vi "COMI PG Change Freq.vi"(9 "freq":dbl, 10 "ch":i32, 11 "hDevice":u32) -> (2 "function return":dbl, 3 "hDevice out":u32)   [LabVIEW 2017, in "Comidll.lvlib"]
doc: "double (COMI_PG_ChangeFreq) (HANDLE hDevice, int ch, double freq);"
uses:
  <userlib>/Comidll/Comidll.lvlib
  <userlib>/Comidll/Comidll.dll
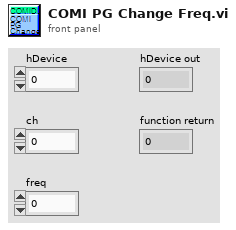
[diagram p1: front panel]
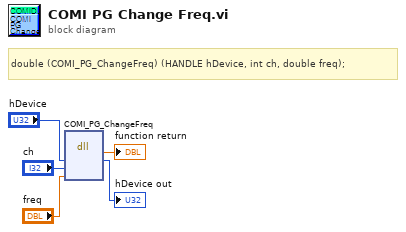
[diagram p0: block diagram]
diagram:
  # "double\t(COMI_PG_ChangeFreq) (HANDLE hDevice, int ch, double freq);"
  n1 = dll-call lib="C:/Program Files/National Instruments/LabVIEW 2017/user.lib/Comidll/Comidll.*" fn="COMI_PG_ChangeFreq"("hDevice"="hDevice", "ch"="ch", "freq"="freq") -> (→"function return":dbl, "hDevice"=→"hDevice out":u32)  [unwired: 5 in, 2 out]
